vi "读取行.vi"(8 "error in (no error)":errorcluster caption="错误输入（无错误）", 11 "串口 输入":refnum<class "串口.lvclass"> caption="DNL_LabVIEW Object in") -> (0 "error out":errorcluster caption="错误输出", 2 "行读取":string, 3 "串口 输出":refnum<class "串口.lvclass"> caption="DNL_LabVIEW Object out")   [LabVIEW 2012, in "串口.lvclass"]
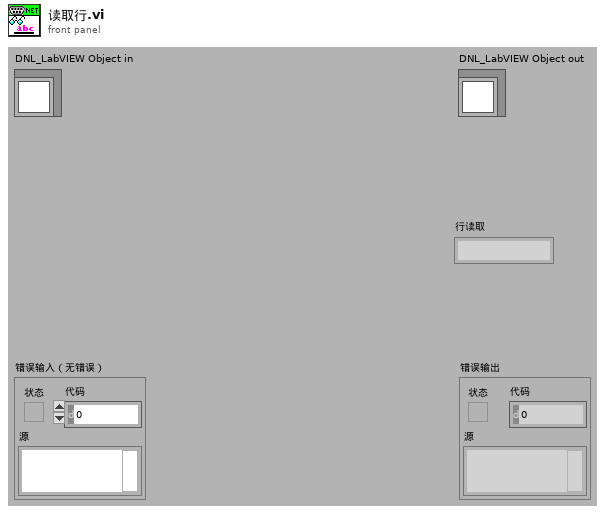
[diagram p1: front panel]
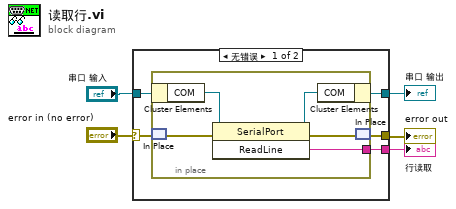
[diagram p0: block diagram]
diagram:
  n1 = case shown="无错误" "error in (no error)" {
    selector: "error in (no error)" -> [w9 w17]
    tunnel: [w8 w17] -> w4
    tunnel: [w6 w16] -> w2
    tunnel: "串口 输入" -> [w10 w16]
    tunnel: [w7 _] -> w1
    frame No Error {
      n2 = in-place {
        in-place-border: [w11] -> w7
        n3 = in-place-cluster #1(w10) -> ("COM"=w15:refnum<k24>)
        n4 = in-place-match #2(w9) -> (w13:errorcluster)
        n5 = invoke class="SerialPort" method="ReadLine"(reference=w15, error in=w13) -> (reference out=w14:refnum<k24>, error out=w12:errorcluster, "ReadLine"=w11:string)  [unwired: 1 in]
        n6 = in-place-cluster #1("COM"=w14) -> (w6:refnum<class "串口.lvclass">)
        n7 = in-place-match #2(w12) -> (w8:errorcluster)
      }
    }
    frame Error {
    }
  }
  "error out" <- w4
  "串口 输出" <- w2
  "行读取" <- w1
